vi "Forward Kinematics (Point).vi"(8 "error in (no error)":errorcluster, 10 "joint positions":dbl[](array[numeric]), 11 "serial arm in":refnum<class "NI_Robotics_Serial Robot Arm.lvclass">) -> (0 "error out":errorcluster, 2 "end effector transform":T1, 3 "serial arm out":refnum<class "NI_Robotics_Serial Robot Arm.lvclass">)   [LabVIEW 2017, in "NI_Kinematics.lvlib"]
doc: "Returns a homogenous transform or transforms that represents the position of a robotic arm end effector given the joint angles of the arm. Wire data to the <B>joint positions</B> input to determine the polymorphic instance to use or manually select the instance.\n\n<B>.m file:</B> fkine"
uses:
  <vilib>/robotics/Kinematics/NI_Kinematics.lvlib
  <vilib>/robotics/Kinematics/Robot/NI_Robotics_Serial Robot Arm.lvclass
  <vilib>/Analysis/Matrix/Datatypes/RealMatrix.ctl
  <vilib>/Analysis/baseanly.llb/Real A x B.vi
  <vilib>/robotics/Kinematics/Link/NI_Robotics_Link.lvclass
  <vilib>/Analysis/NI_AALBase.lvlib
  <vilib>/robotics/Utilities/NI_Robotics Utilities.lvlib
  <vilib>/Analysis/Matrix/NI_Matrix.lvlib
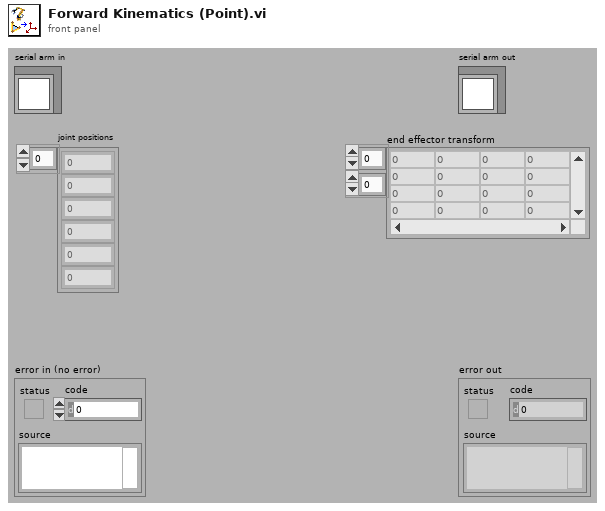
[diagram p1: front panel]
types:
  T1 = typedef "NI_Matrix.lvlib/RealMatrix.ctl" = dbl[][]
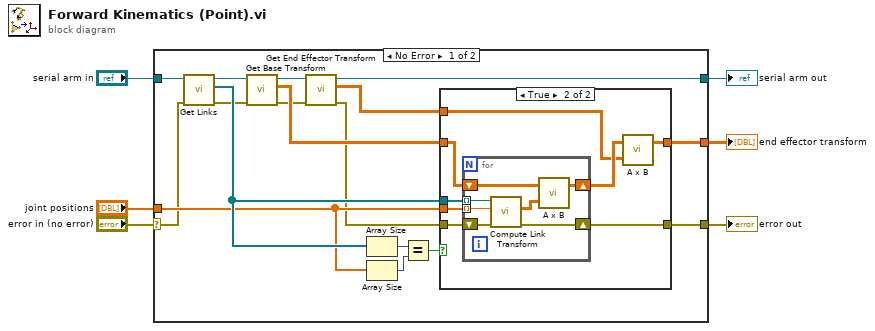
[diagram p0: block diagram]
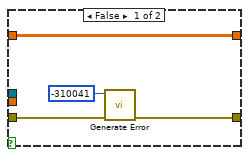
[diagram p2: hidden frame]
diagram:
  n1 = case shown="No Error" "error in (no error)" {
    selector: "error in (no error)" -> [w8 w44]
    tunnel: [w23 w44] -> w5
    tunnel: [w9 w43] -> w3
    tunnel: "serial arm in" -> [w14 w43]
    tunnel: "joint positions" -> [w18 _]
    tunnel: [w22 _] -> w1
    frame No Error {
      n2 = call <vilib>:"Get Links.vi"("error in (no error)"=w8, "serial arm in"=w14) -> ("error out"=w12:errorcluster, "links"=w19:refnum<class "NI_Robotics_Link.lvclass">[], "serial arm out"=w13:refnum<class "NI_Robotics_Serial Robot Arm.lvclass">)  [unwired: 7 in]
      n3 = call <vilib>:"Get Base Transform.vi"("error in (no error)"=w12, "serial arm in"=w13) -> ("error out"=w10:errorcluster, "base transform"=w20:T1, "serial arm out"=w11:refnum<class "NI_Robotics_Serial Robot Arm.lvclass">)  [unwired: 7 in]
      n4 = call <vilib>:"Get End Effector Transform.vi"("error in (no error)"=w10, "serial arm in"=w11) -> ("error out"=w7:errorcluster, "end effector transform"=w21:T1, "serial arm out"=w9:refnum<class "NI_Robotics_Serial Robot Arm.lvclass">)  [unwired: 7 in]
      n5 = Array Size(array=w19) -> (size(s)=w16:i32)
      n6 = Array Size(array=w18) -> (size(s)=w17:i32)
      n7 = Equal?(x=w16, y=w17) -> (x = y?=w15:bool)
      n8 = case shown="True" w15 {
        tunnel: [w25 w35] -> w23
        tunnel: [w27 w34] -> w22
        tunnel: w7 -> [w26 w32]
        tunnel: w21 -> [_ w31]
        tunnel: w20 -> [w27 w30]
        tunnel: w19 -> [_ w29]
        tunnel: w18 -> [_ w28]
        frame False {
          n9 = call <vilib>:"Generate Error.vi"("error in (no error)"=w26, "code"=-310041) -> ("error out"=w25:errorcluster)  [unwired: 9 in]
        }
        frame True {
          n10 = for {
            tunnel: w29 -> [w42] mode=indexing
            shift-right: [w36] -> w33
            shift-left: w30 -> [w38]
            tunnel: w28 -> [w41] mode=indexing
            shift-right: [w40] -> w35
            shift-left: w32 -> [w39]
            n11 = call <vilib>:"Compute Link Transform.vi"("error in (no error)"=w39, "q"=w41, "Link in"=w42) -> ("error out"=w40:errorcluster, "Link Transform"=w37:T1)  [unwired: 7 out]
            n12 = call-poly <vilib>:"A x B.vi"("B"=w37, "A"=w38) -> ("A x B"=w36:T1)  [unwired: 1 out]
          }
          n13 = call-poly <vilib>:"A x B.vi"("B"=w31, "A"=w33) -> ("A x B"=w34:T1)  [unwired: 1 out]
        }
      }
    }
    frame Error {
    }
  }
  "error out" <- w5
  "serial arm out" <- w3
  "end effector transform" <- w1
